vi "To Serial Form.vi"(6 "Serial Version":T1, 10 "Serializer in":refnum<class "Serializer.lvclass">, 11 "Data in":refnum<class "Data.lvclass">) -> (0 "error out":errorcluster, 2 "Serializer out":refnum<class "Serializer.lvclass">, 3 "Data out":refnum<class "Data.lvclass">)   [LabVIEW 2014, in "Base Data Class.lvlib" / "Data.lvclass"]
uses:
  Data.lvclass
  <vilib>/NI/AQ Character Lineator/Serializer/Serializer.lvclass
  <vilib>/NI/AQ Character Lineator/Serialization Common/Serial Version.ctl
  Data.lvclass/Data.ctl
  <vilib>/NI/AQ Character Lineator/Serializable/Insert Timestamp.vi
  <vilib>/NI/AQ Character Lineator/Serializer/Insert Timestamp.vi
  <vilib>/NI/AQ Character Lineator/Serializer/Read Include Default Values.vi
  <vilib>/NI/AQ Character Lineator/Serializable/Serializable.lvclass
  <vilib>/NI/AQ Character Lineator/Serialization Common/Serialization Common.lvlib
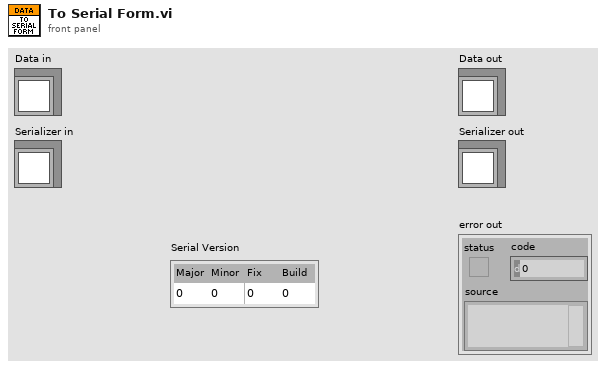
[diagram p1: front panel]
types:
  T1 = typedef "Serialization Common.lvlib/Serial Version.ctl" = cluster{"Major":u16, "Minor":u16, "Fix":u16, "Build":u16}
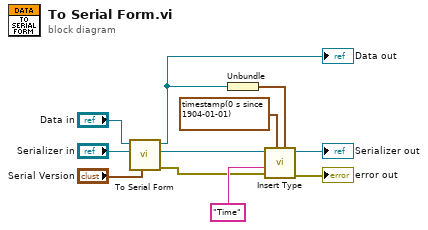
[diagram p0: block diagram]
diagram:
  n1 = call-parent "To Serial Form.vi"("Serial Version"="Serial Version", "Serializer in"="Serializer in", "Serializable in"="Data in") -> ("error out"=w4:errorcluster, "Serializer out"=w7:refnum<class "Serializer.lvclass">, "Serializable out"=w1:refnum<class "Data.lvclass">)  [unwired: 6 in]
  "Data out" <- w1
  n2 = Unbundle(w1) -> (w2:timestamp)
  n3 = call-poly <vilib>:"Insert Type.vi"("Time Stamp"=w2, "Default Value"=timestamp(0 s since 1904-01-01), "error in (no error)"=w4, "Name"="Time", "Serializer in"=w7) -> ("error out"=→"error out":errorcluster, "Serializer out"=→"Serializer out":refnum<class "Serializer.lvclass">)  [unwired: 5 in]
